vi "Create Error Cluster.vi"(8 "error in (no error)":errorcluster, 11 "front panel":refnum<vi>) -> (0 "error out":errorcluster, 2 "error in/out control":refnum<vi>[](array[refnum]), 3 "front panel out":refnum<vi>)   [LabVIEW 2018, in "NISAST VI Scripting.lvlib" / "VI.lvlib" / "Front Panel.lvlib"]
uses:
  Front Panel.lvlib
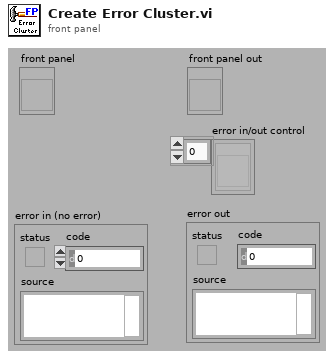
[diagram p1: front panel]
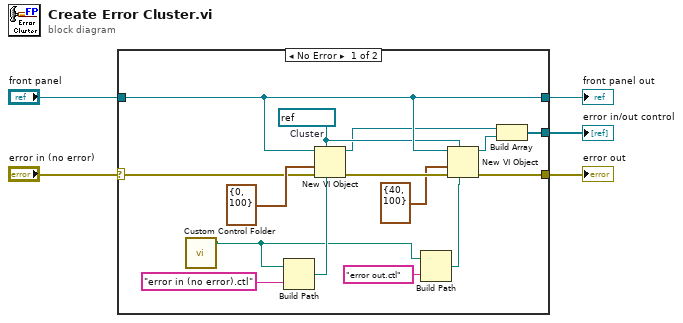
[diagram p0: block diagram]
diagram:
  n1 = case shown="No Error" "error in (no error)" {
    selector: "error in (no error)" -> [w17 w22]
    tunnel: [w15 w22] -> w4
    tunnel: "front panel" -> [w14 w21]
    tunnel: [w14 w21] -> w2
    tunnel: [w7 _] -> w1
    frame No Error {
      w13 = refnum<vi> refnum  # Cluster
      n2 = call "Custom Control Folder.vi"() -> ("custom control folder out"=w6:path)  [unwired: 2 in, 9 out]
      n3 = Build Path(base path=w6, name or relative path="error in (no error).ctl") -> (appended path=w18:path)
      n4 = New VI Object(vi object class=w13, owner refnum=w14, position/next to=cluster{"Horizontal":i16, "Vertical":i16} {"Horizontal"=0, "Vertical"=100}, 6:w18, 8:w17) -> (object refnum=w9:refnum<vi>, 0:w16:errorcluster)  [unwired: 3 out]
      n5 = Build Path(base path=w6, name or relative path="error out.ctl") -> (appended path=w10:path)
      n6 = New VI Object(vi object class=w13, owner refnum=w14, position/next to=cluster{"Horizontal":i16, "Vertical":i16} {"Horizontal"=40, "Vertical"=100}, 6:w10, 8:w16) -> (object refnum=w8:refnum<vi>, 0:w15:errorcluster)  [unwired: 3 out]
      n7 = Build Array(w9, w8) -> (w7:refnum<vi>[])
    }
    frame Error {
    }
  }
  "error out" <- w4
  "front panel out" <- w2
  "error in/out control" <- w1
